vi "Pre Launch Init.vi"(11 "SensorView in":refnum<class "SensorView.lvclass">) -> (0 "error out":errorcluster, 3 "SensorView out":refnum<class "SensorView.lvclass">)   [LabVIEW 2012, in "Sensor Definition.lvlib" / "SensorView.lvclass"]
doc: "(<B>Filename</B>: Actor Framework.lvlib:Actor.lvclass:Pre Launch Init.vi)\n\nDefines behavior that occurs after the Launch Actor method is invoked but before the actor's Actor Core method begins running.\n\nThe Pre Launch Init method is guaranteed to finish before the Launch Actor method returns to its caller and before the actor itself receives any messages. Any references that the Pre Launch Init method obtains are guaranteed to have the same lifetime as the actor itself. Any errors that the Pre Launch Init method returns will abort the launch.\n\nBy default, this method does nothing. A descendant class may override it to define behavior."
uses:
  SensorView.lvclass
  SensorInfo.lvclass
  SensorData.lvclass
  SensorView.lvclass/SensorView.ctl
  Win8uiFramework/ViewableActor.lvclass
  Write SensorInfo Changed Event.vi
  Write SensorData Changed Event.vi
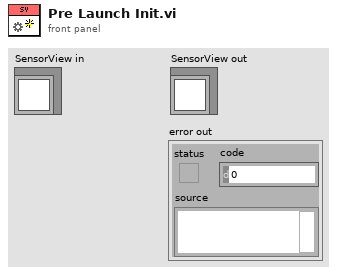
[diagram p1: front panel]
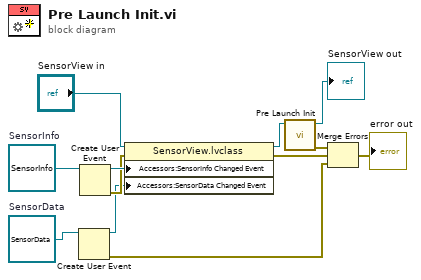
[diagram p0: block diagram]
diagram:
  w3 = refnum<class "SensorData.lvclass"> refnum  # SensorData
  w10 = refnum<class "SensorInfo.lvclass"> refnum  # SensorInfo
  n1 = Create User Event(user event datatype=w3) -> (user event=w2:refnum<user-event>, error out=w1:errorcluster)  [unwired: 1 in]
  n2 = Create User Event(user event datatype=w10) -> (user event=w8:refnum<user-event>, error out=w7:errorcluster)  [unwired: 1 in]
  n3 = property class="SensorView.lvclass"(reference="SensorView in", error in=w7, "Accessors:SensorInfo Changed Event"=w8, "Accessors:SensorData Changed Event"=w2) -> (reference out=w9:refnum<class "SensorView.lvclass">, error out=w5:errorcluster)
  n4 = call-parent "Pre Launch Init.vi"("ViewableActor in"=w9) -> ("error out"=w6:errorcluster, "ViewableActor out"=→"SensorView out":refnum<class "SensorView.lvclass">)  [unwired: 9 in]
  n5 = Merge Errors(w6, w5, w1) -> (→"error out":errorcluster)
